vi "Subvi timeout.vi"(8 "Timeout":i16, 10 "Input":bool) -> (2 "Output":bool)   [LabVIEW 2017]
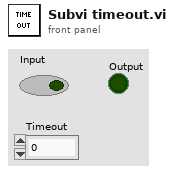
[diagram p1: front panel]
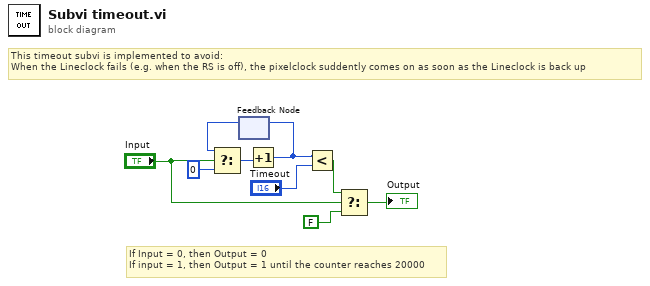
[diagram p0: block diagram]
diagram:
  # "This timeout subvi is implemented to avoid:\nWhen the Lineclock fails (e.g. when the RS is off), the pixelclock suddently comes on as soon as the Lineclock is back up"
  # "If Input = 0, then Output = 0\nIf input = 1, then Output = 1 until the counter reaches 20000"
  n1 = feedback #1() -> (w9:i16)  [unwired: 1 in]
  n2 = Select(t=w9, s="Input", f=i16 0) -> (s? t:f=w8:i16)
  n3 = Increment(x=w8) -> (x+1=w4:i16)
  n4 = feedback-in #1(w4) -> ()
  n5 = Less?(x=w4, y="Timeout") -> (x < y?=w6:bool)
  n6 = Select(t=w6, s="Input", f=FALSE) -> (s? t:f=→"Output":bool)
